vi "Read Response Headers.vi"(8 "error in (no error)":errorcluster, 11 "HttpResponseMessage in":refnum<class "HttpResponseMessage.lvclass">) -> (0 "error out":errorcluster, 2 "HTTPHeaders_NET out":refnum<class "HttpHeaders_Response.lvclass">, 3 "HttpResponseMessage out":refnum<class "HttpResponseMessage.lvclass">)   [LabVIEW 2018, in "HttpClient_NET.lvlib" / "HttpResponseMessage.lvclass"]
doc: "<b> </b> <b> </b>\nHttpClient_NET\nJustin Young - Viviota\nCopyright (c) 2021\nLicense: BSD"
uses:
  HttpResponseMessage.lvclass
  HttpHeaders_response/HttpHeaders_Response.lvclass
  C:/Viviota/Projects/R&D/LabVIEW_HTTP_REST_NET/HTTPHeaders_NET/HttpHeaders_NET.lvclass
  HttpResponseMessage.lvclass/HttpResponseMessage.ctl
  System.Net.Http
  Accessors/Write HttpHeaders_Response.vi
  Accessors/Read NET_HttpReponseMessage.vi
  Accessors/Read HttpHeaders_Response.vi
  HTTPHeaders_NET/HttpHeaders_NET.lvclass
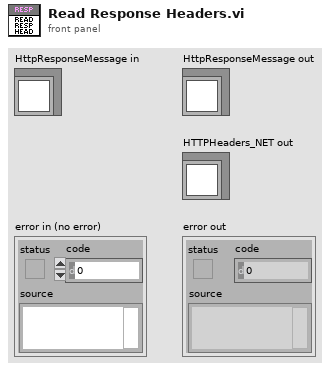
[diagram p1: front panel]
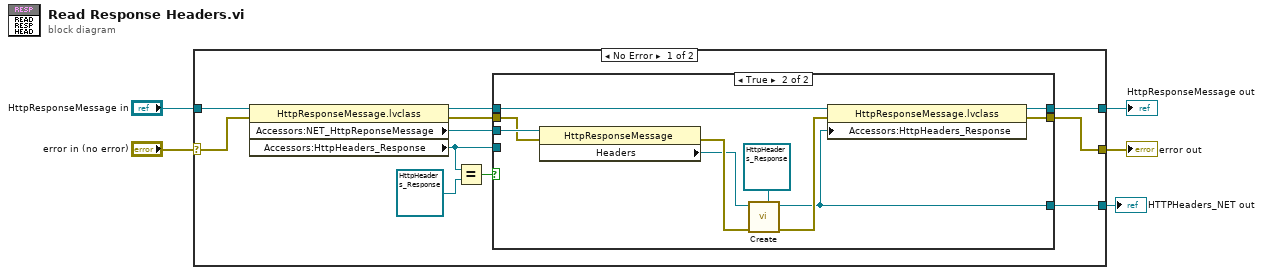
[diagram p0: block diagram]
diagram:
  n1 = case shown="No Error" "error in (no error)" {
    selector: "error in (no error)" -> [w16 w31]
    tunnel: [w11 w31] -> w4
    tunnel: [w9 w30] -> w2
    tunnel: "HttpResponseMessage in" -> [w15 w30]
    tunnel: [w12 _] -> w1
    frame No Error {
      n2 = property class="HttpResponseMessage.lvclass"(reference=w15, error in=w16) -> (reference out=w10:refnum<class "HttpResponseMessage.lvclass">, error out=w13:errorcluster, "Accessors:NET_HttpReponseMessage"=w14:refnum<k24>, "Accessors:HttpHeaders_Response"=w6:refnum<class "HttpHeaders_Response.lvclass">)
      n3 = Equal?(x=w6, y=refnum<class "HttpHeaders_Response.lvclass"> refnum) -> (x = y?=w7:bool)
      n4 = case shown="True" w7 {
        tunnel: w14 -> [_ w29]
        tunnel: w13 -> [w17 w28]
        tunnel: [w19 w20] -> w12
        tunnel: [w17 w23] -> w11
        tunnel: w10 -> [w18 w22]
        tunnel: [w18 w21] -> w9
        tunnel: w6 -> [w19 _]
        frame False {
        }
        frame True {
          n5 = property class="HttpResponseMessage"(reference=w29, error in=w28) -> (error out=w27:errorcluster, "Headers"=w24:refnum<k24>)  [unwired: 1 out]
          n6 = call "Create.vi"("HTTPHeaders_NET in"=refnum<class "HttpHeaders_Response.lvclass"> refnum ("LabVIEWHTTPClient_NET.lvlib:HttpHeaders_Response.lvclass"), "error in (no error)"=w27, "NET_HttpHeaders"=w24) -> ("error out"=w26:errorcluster, "HTTPHeaders_NET out"=w20:refnum<class "HttpHeaders_Response.lvclass">)  [unwired: 7 in]
          n7 = property class="HttpResponseMessage.lvclass"(reference=w22, error in=w26, "Accessors:HttpHeaders_Response"=w20) -> (reference out=w21:refnum<class "HttpResponseMessage.lvclass">, error out=w23:errorcluster)
        }
      }
    }
    frame Error {
    }
  }
  "error out" <- w4
  "HttpResponseMessage out" <- w2
  "HTTPHeaders_NET out" <- w1
